vi "PS4 Controller - Event Read.vi"() -> ()   [LabVIEW 2011, in "LVH-PS4.lvlib"]
doc: "This example demonstrates how to read from a Play Station 4 controller using events."
uses:
  vi.lib/LabVIEW Hacker/PS4-Controller/LVH-PS4.lvlib
  vi.lib/LabVIEW Hacker/PS4-Controller/Private/Type Defs/Axis.ctl
  vi.lib/LabVIEW Hacker/PS4-Controller/Private/Type Defs/Indicators/DPad Enum.ctl
panel:
  out "All Axis":T1
  out "Event Log":string[](array[string])
  in  "Device Index":i32
  in  "Stop Button":bool
  # "PS4 Controller  - Event Based Read\n\nThis example demonstrates how to read all buttons and axis data from an PS4 controller using events.\n\nInstructions\n1. Select the Device Index associated with the PS4 Controller.\n2. Click the Run Arrow.\n3. Notice the controller data on the front panel update to match the actual controller state."
  # "Configure"
  # "Controller Data"
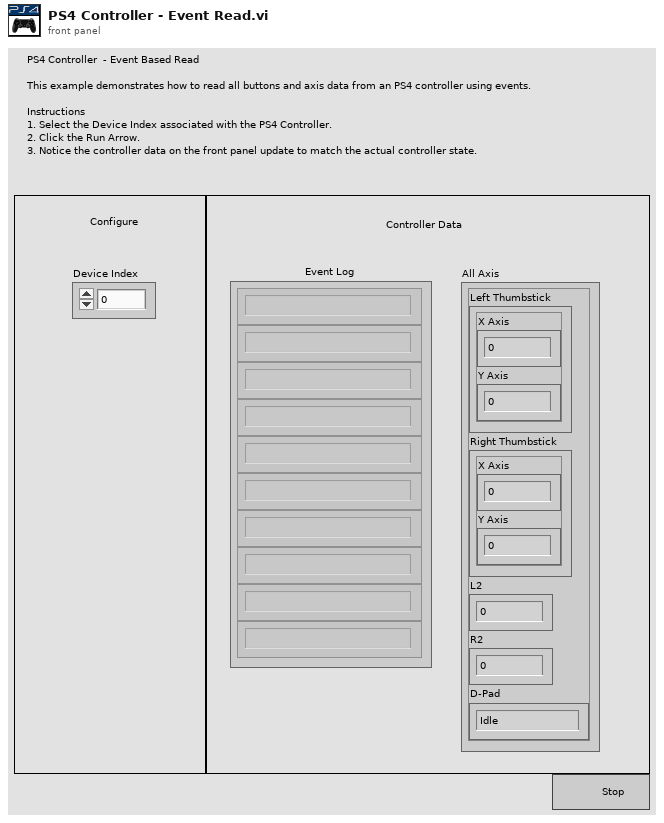
[diagram p1: front panel]
types:
  T1 = typedef "LVH-PS4.lvlib/Axis.ctl" = cluster{"Left Thumbstick":cluster{"X Axis":i32, "Y Axis":i32}, "Right Thumbstick":cluster{"X Axis":i32, "Y Axis":i32}, "L2":i32, "R2":i32, "D-Pad":T2}
  T2 = typedef "LVH-PS4.lvlib/DPad Enum.ctl" = enum16{"Idle", "Up", "Up / Right", "Right", "Down / Right", "Down", "Down / Left", "Left", "Up / Left"}
  T3 = typedef "LVH-PS4.lvlib/PS4 Controller Ref.ctl" = cluster{"Controller Ref":refnum<k1>, "PS4 Events Ref":refnum<event-registration>, "Worker Ref":refnum<vi>}
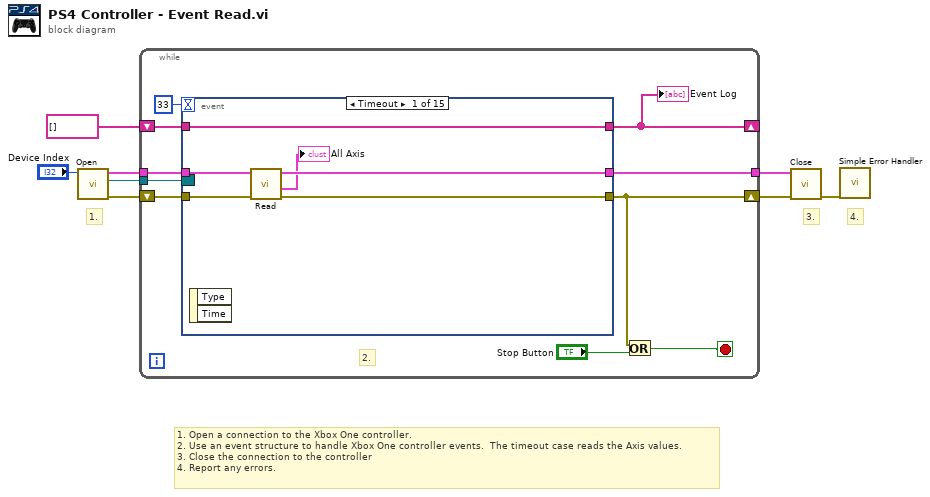
[diagram p0: block diagram]
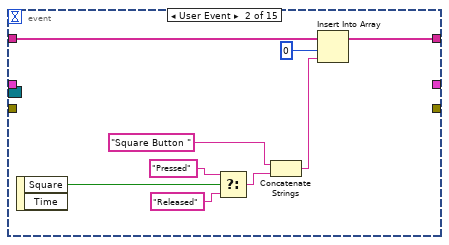
[diagram p2: hidden frame]
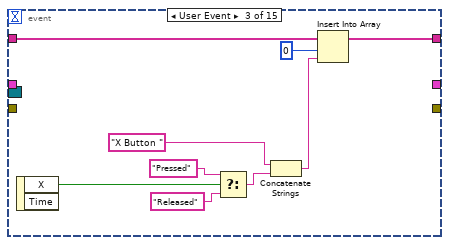
[diagram p3: hidden frame]
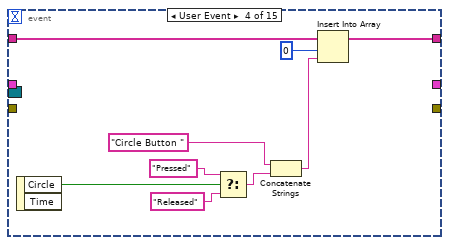
[diagram p4: hidden frame]
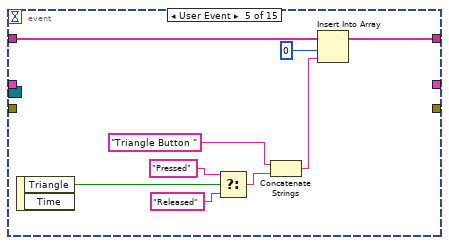
[diagram p5: hidden frame]
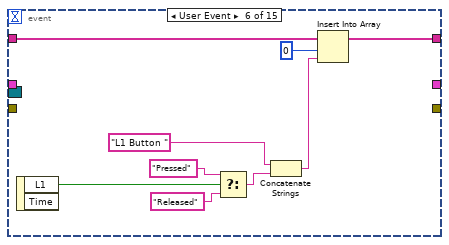
[diagram p6: hidden frame]
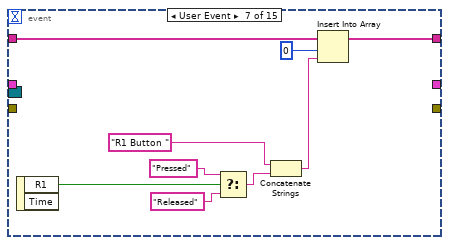
[diagram p7: hidden frame]
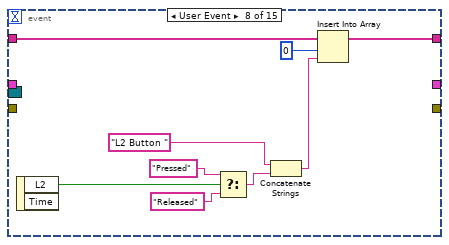
[diagram p8: hidden frame]
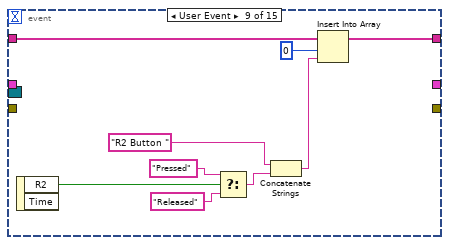
[diagram p9: hidden frame]
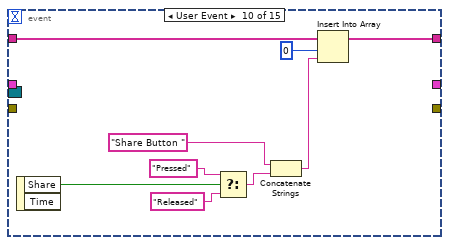
[diagram p10: hidden frame]
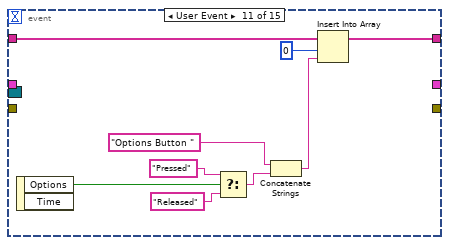
[diagram p11: hidden frame]
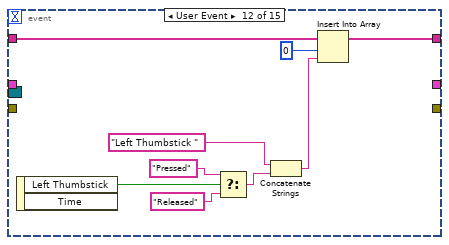
[diagram p12: hidden frame]
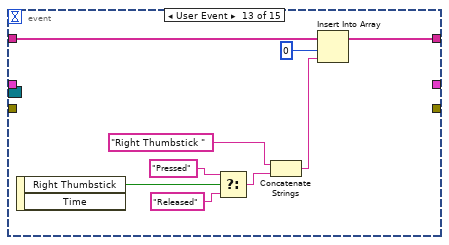
[diagram p13: hidden frame]
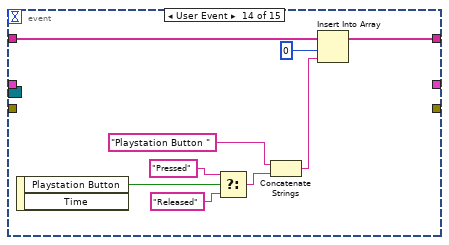
[diagram p14: hidden frame]
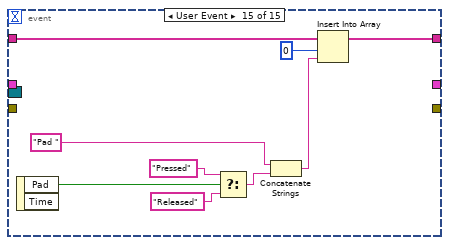
[diagram p15: hidden frame]
diagram:
  # "4."
  # "3."
  # "1."
  # "1. Open a connection to the Xbox One controller.\n2. Use an event structure to handle Xbox One controller events.  The timeout case reads the Axis values.\n3. Close the connection to the controller\n4. Report any errors."
  n1 = call "Open.vi"("Device Index"="Device Index") -> ("Error Out"=w6:errorcluster, "PS4 Event Refs"=w4:refnum<event-registration>, "PS4 Controller Ref"=w5:T3)  [unwired: 8 in]
  n2 = while {
    shift-right: [w14] -> w8
    shift-left: w6 -> [w17]
    tunnel: w5 -> [w18]
    tunnel: [w13] -> w7
    tunnel: w4 -> [w11]
    shift-right: [w9] -> _
    shift-left: string[] [] ("Event Log") -> [w10]
    stop <- w16 stop-if-true
    # "2."
    n3 = event shown="[0] Timeout" {
      selector: w11 -> [_ _ _ _ _ _ _ _ _ _ _ _ _ _ _]
      dyn-events: _ -> [_ _ _ _ _ _ _ _ _ _ _ _ _ _ _]
      timeout: 33 -> [_ _ _ _ _ _ _ _ _ _ _ _ _ _ _]
      tunnel: w18 -> [w23 _ _ _ _ _ _ _ _ _ _ _ _ _ _]
      tunnel: w17 -> [w22 _ _ _ _ _ _ _ _ _ _ _ _ _ _]
      tunnel: [w21 _ _ _ _ _ _ _ _ _ _ _ _ _ _] -> w14
      tunnel: [w20 _ _ _ _ _ _ _ _ _ _ _ _ _ _] -> w13
      tunnel: w10 -> [w24 w33 w42 w51 w60 w69 w78 w87 w96 w105 w114 w123 w132 w141 w150]
      tunnel: [w24 w25 w34 w43 w52 w61 w70 w79 w88 w97 w106 w115 w124 w133 w142] -> w9
      event Timeout {
        n4 = event-data() -> ()  [unwired: 1 in, 2 out]
        n5 = call "Read.vi"("Error In"=w22, "PS4 Controller Ref"=w23) -> ("Error Out"=w21:errorcluster, "All Axis"=→"All Axis":T1, "PS4 Controller Ref"=w20:T3)  [unwired: 6 in, 1 out]
      }
      event User Event {
        n6 = event-data() -> ("Square"=w32:bool)  [unwired: 1 in, 1 out]
        n7 = Select(t="Pressed", s=w32, f="Released") -> (s? t:f=w30:string)
        n8 = Concatenate Strings("Square Button ", w30) -> (w27:string)
        n9 = Insert Into Array(array=w33, index=0, new element=w27) -> (w25:string[])
      }
      event User Event {
        n10 = event-data() -> ("X"=w41:bool)  [unwired: 1 in, 1 out]
        n11 = Select(t="Pressed", s=w41, f="Released") -> (s? t:f=w39:string)
        n12 = Concatenate Strings("X Button ", w39) -> (w36:string)
        n13 = Insert Into Array(array=w42, index=0, new element=w36) -> (w34:string[])
      }
      event User Event {
        n14 = event-data() -> ("Circle"=w50:bool)  [unwired: 1 in, 1 out]
        n15 = Select(t="Pressed", s=w50, f="Released") -> (s? t:f=w48:string)
        n16 = Concatenate Strings("Circle Button ", w48) -> (w45:string)
        n17 = Insert Into Array(array=w51, index=0, new element=w45) -> (w43:string[])
      }
      event User Event {
        n18 = event-data() -> ("Triangle"=w59:bool)  [unwired: 1 in, 1 out]
        n19 = Select(t="Pressed", s=w59, f="Released") -> (s? t:f=w57:string)
        n20 = Concatenate Strings("Triangle Button ", w57) -> (w54:string)
        n21 = Insert Into Array(array=w60, index=0, new element=w54) -> (w52:string[])
      }
      event User Event {
        n22 = event-data() -> ("L1"=w68:bool)  [unwired: 1 in, 1 out]
        n23 = Select(t="Pressed", s=w68, f="Released") -> (s? t:f=w66:string)
        n24 = Concatenate Strings("L1 Button ", w66) -> (w63:string)
        n25 = Insert Into Array(array=w69, index=0, new element=w63) -> (w61:string[])
      }
      event User Event {
        n26 = event-data() -> ("R1"=w77:bool)  [unwired: 1 in, 1 out]
        n27 = Select(t="Pressed", s=w77, f="Released") -> (s? t:f=w75:string)
        n28 = Concatenate Strings("R1 Button ", w75) -> (w72:string)
        n29 = Insert Into Array(array=w78, index=0, new element=w72) -> (w70:string[])
      }
      event User Event {
        n30 = event-data() -> ("L2"=w86:bool)  [unwired: 1 in, 1 out]
        n31 = Select(t="Pressed", s=w86, f="Released") -> (s? t:f=w84:string)
        n32 = Concatenate Strings("L2 Button ", w84) -> (w81:string)
        n33 = Insert Into Array(array=w87, index=0, new element=w81) -> (w79:string[])
      }
      event User Event {
        n34 = event-data() -> ("R2"=w95:bool)  [unwired: 1 in, 1 out]
        n35 = Select(t="Pressed", s=w95, f="Released") -> (s? t:f=w93:string)
        n36 = Concatenate Strings("R2 Button ", w93) -> (w90:string)
        n37 = Insert Into Array(array=w96, index=0, new element=w90) -> (w88:string[])
      }
      event User Event {
        n38 = event-data() -> ("Share"=w104:bool)  [unwired: 1 in, 1 out]
        n39 = Select(t="Pressed", s=w104, f="Released") -> (s? t:f=w102:string)
        n40 = Concatenate Strings("Share Button ", w102) -> (w99:string)
        n41 = Insert Into Array(array=w105, index=0, new element=w99) -> (w97:string[])
      }
      event User Event {
        n42 = event-data() -> ("Options"=w113:bool)  [unwired: 1 in, 1 out]
        n43 = Select(t="Pressed", s=w113, f="Released") -> (s? t:f=w111:string)
        n44 = Concatenate Strings("Options Button ", w111) -> (w108:string)
        n45 = Insert Into Array(array=w114, index=0, new element=w108) -> (w106:string[])
      }
      event User Event {
        n46 = event-data() -> ("Left Thumbstick"=w122:bool)  [unwired: 1 in, 1 out]
        n47 = Select(t="Pressed", s=w122, f="Released") -> (s? t:f=w120:string)
        n48 = Concatenate Strings("Left Thumbstick ", w120) -> (w117:string)
        n49 = Insert Into Array(array=w123, index=0, new element=w117) -> (w115:string[])
      }
      event User Event {
        n50 = event-data() -> ("Right Thumbstick"=w131:bool)  [unwired: 1 in, 1 out]
        n51 = Select(t="Pressed", s=w131, f="Released") -> (s? t:f=w129:string)
        n52 = Concatenate Strings("Right Thumbstick ", w129) -> (w126:string)
        n53 = Insert Into Array(array=w132, index=0, new element=w126) -> (w124:string[])
      }
      event User Event {
        n54 = event-data() -> ("Playstation Button"=w140:bool)  [unwired: 1 in, 1 out]
        n55 = Select(t="Pressed", s=w140, f="Released") -> (s? t:f=w138:string)
        n56 = Concatenate Strings("Playstation Button ", w138) -> (w135:string)
        n57 = Insert Into Array(array=w141, index=0, new element=w135) -> (w133:string[])
      }
      event User Event {
        n58 = event-data() -> ("Pad"=w149:bool)  [unwired: 1 in, 1 out]
        n59 = Select(t="Pressed", s=w149, f="Released") -> (s? t:f=w147:string)
        n60 = Concatenate Strings("Pad ", w147) -> (w144:string)
        n61 = Insert Into Array(array=w150, index=0, new element=w144) -> (w142:string[])
      }
    }
    "Event Log" <- w9
    n62 = Or(x=w14, y="Stop Button") -> (x .or. y?=w16:bool)
  }
  n63 = call "Close.vi"("Error In"=w8, "PS4 Controller Ref"=w7) -> ("Error Out"=w1:errorcluster)  [unwired: 9 in]
  n64 = call <vilib>:"Simple Error Handler.vi"("error in (no error)"=w1) -> ()  [unwired: 4 in, 5 out]
